vi "Read UI.vi"(8 "error in (no error)":errorcluster, 11 "Chef State in":refnum<class "Chef State.lvclass">) -> (0 "error out":errorcluster, 2 "UI":refnum<class "Message Enqueuer.lvclass">, 3 "Chef State out":refnum<class "Chef State.lvclass">)   [LabVIEW 2024, in "Chef State.lvlib" / "Chef State.lvclass"]
uses:
  Chef State.lvclass
  Chef State.lvclass/Chef State.ctl
  <vilib>/ActorFramework/Message Enqueuer/Message Enqueuer.lvclass
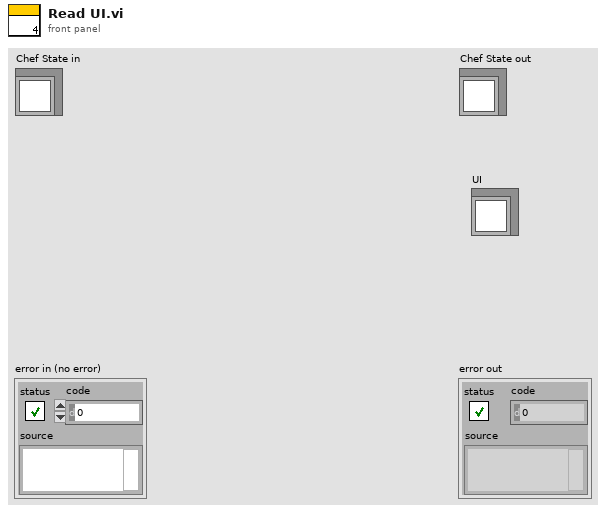
[diagram p1: front panel]
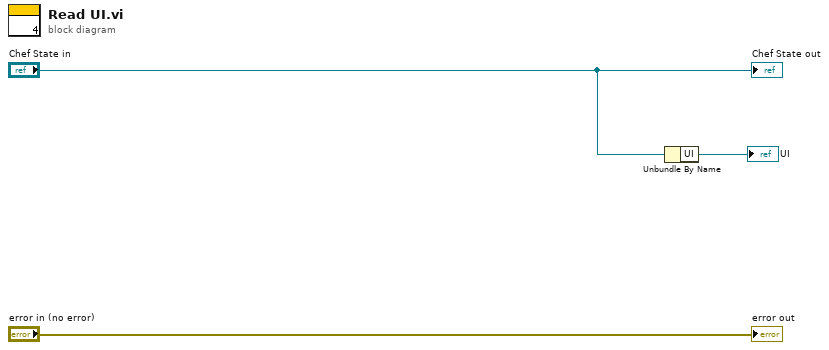
[diagram p0: block diagram]
diagram:
  n1 = Unbundle By Name("Chef State in") -> ("UI"=→"UI":refnum<class "Message Enqueuer.lvclass">)
  "error out" <- "error in (no error)"
  "Chef State out" <- "Chef State in"
